vi "Initialize Input DMA Refs.vi"(8 "error in (no error)":errorcluster, 10 "Settings.Compiled":T1 {"IncomingRegisters.Settings"."Register"."Data Type" format="%.0x"; "IncomingRegisters.Refs"."Refs"."Data Reference" format="%.0x"; "OutgoingRegisters.Settings"."Register"."Data Type" format="%.0x"; "OutgoingRegisters.Refs"."Refs"."Data Reference" format="%.0x"; "IncomingDMA.Settings"."DMA.Settings"."DMA Host Buffer" items=["1 Second"=1, "2 Seconds"=2, "5 Seconds"=5, "10 Seconds"=10]; "IncomingDMA.Settings"."DMA.Settings"."dt" format="%#_p"; "IncomingDMA.Settings"."DMA.Settings"."Update Rate" items=["1 Hz"=1, "2 Hz"=2, "5 Hz"=5, "10 Hz"=10]; "OutgoingDMA.Settings"."DMA.Settings"."DMA Host Buffer" items=["1 Second"=1, "2 Seconds"=2, "5 Seconds"=5, "10 Seconds"=10]; "OutgoingDMA.Settings"."DMA.Settings"."dt" format="%#_p"; "OutgoingDMA.Settings"."DMA.Settings"."Update Rate" items=["1 Hz"=1, "2 Hz"=2, "5 Hz"=5, "10 Hz"=10]}, 11 "FPGA Ref":refnum<k20>) -> (0 "error out":errorcluster, 2 "DMA Settings":T15[](array[typedef]) {"DMA Settings"."DMA Host Buffer" items=["1 Second"=1, "2 Seconds"=2, "5 Seconds"=5, "10 Seconds"=10]; "DMA Settings"."dt" format="%#_p"; "DMA Settings"."Update Rate" items=["1 Hz"=1, "2 Hz"=2, "5 Hz"=5, "10 Hz"=10]}, 3 "FPGA Ref":refnum<k20>)   [LabVIEW 2016, in "FPGA Addon Engine.lvlib"]
uses:
  FPGA Addon Engine.lvlib
  Types/DMA Input References.ctl
  <vilib>/NI Veristand/Custom Device Waveform API/Multiple Waveforms Write (DBL)/Multiple Waveforms Write (DBL).lvclass
  Types/DMA Input Ref.ctl
  FPGA-Resource-Manager-APIs/Source/Shared/Types/DMA Settings.ctl
  FPGA-Resource-Manager-APIs/Source/Shared/Types/Delacing Scheme.ctl
  FPGA-Resource-Manager-APIs/Source/Shared/Types/DMA Acquisition Mode.ctl
  FPGA-Resource-Manager-APIs/Source/Shared/Types/Compiled.Settings.ctl
  FPGA-Resource-Manager-APIs/Source/Shared/Types/Compiled.RegisterSettings.ctl
  FPGA-Resource-Manager-APIs/Source/Shared/Types/Scalar Type.ctl
  FPGA-Resource-Manager-APIs/Source/Shared/Types/Register Information.ctl
  FPGA-Resource-Manager-APIs/Source/Shared/Types/Data Type.ctl
  <vilib>/NI Veristand/Custom Device API/Block Data Reference.ctl
  <vilib>/NI Veristand/Custom Device API/Data Reference.ctl
  FPGA-Resource-Manager-APIs/Source/Shared/Types/Compiled.DMASettings.ctl
  <vilib>/NI Veristand/Custom Device API/Waveform Data Reference.ctl
  FPGA-Resource-Manager-APIs/Source/Shared/Types/FPGA Settings.ctl
  <vilib>/NI Veristand/Custom Device API/Custom Device Target Type.ctl
  <vilib>/NI/LVFPGA Adv Session Resources/OpenByNameSubVI.vi
  <vilib>/NI Veristand/Custom Device Waveform API/Multiple Waveforms Write (DBL)/NI VeriStand - Open Multiple Waveforms Write Session (DBL).vi
  <vilib>/Utility/error.llb/Error Cluster From Error Code.vi
  <vilib>/rvi/interface/common/niFpgaWaitOnOcc.vi
  <vilib>/rvi/interface/common/dynamic/niFpgaEscapeDelimiterAndNull.vi
  <vilib>/rvi/interface/nirviMethod/nirviMethod.xnode
  <vilib>/NI/LVFPGA Adv Session Resources/OpenByName.xnode
  <vilib>/NI VeriStand/Custom Device Waveform API/NI_VS Custom Device Waveform API.lvlib
  <vilib>/rvi/errors/niLvFpgaMergeErrorWithErrorCode.vi
  FPGA-Resource-Manager-APIs/Source/Shared/FPGA RM Shared API.lvlib
  <vilib>/FPGAPlugInAG/Dynamic/niLvFpga_ConfigureFifo_Dynamic.vi
  <vilib>/FPGAPlugInAG/Dynamic/niLvFpga_StartFifo_Dynamic.vi
  <vilib>/NI/LVFPGA Adv Session Resources/LVFPGAAdvSessionResources.lvlib
  <vilib>/NI VeriStand/Custom Device API/Custom Device API.lvlib
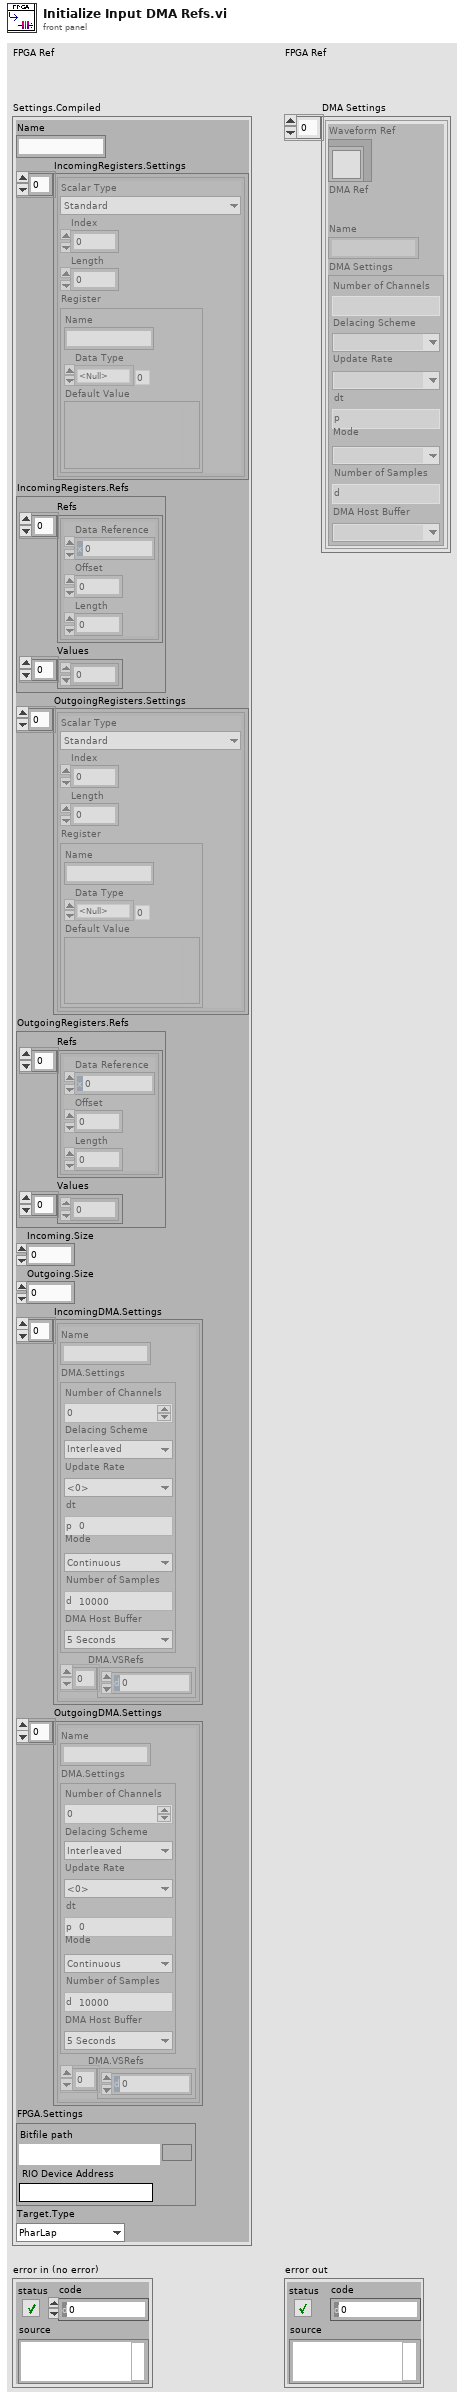
[diagram p1: front panel]
types:
  T1 = typedef "FPGA RM Shared API.lvlib/Compiled.Settings.ctl" = cluster{"Name":string, "IncomingRegisters.Settings":T2[], "IncomingRegisters.Refs":cluster{"Refs":T6[], "Values":dbl[]}, "OutgoingRegisters.Settings":T2[], "OutgoingRegisters.Refs":cluster{"Refs":T6[], "Values":dbl[]}, "Incoming.Size":i32, "Outgoing.Size":i32, "IncomingDMA.Settings":T8[], "OutgoingDMA.Settings":T8[], "FPGA.Settings":T13, "Target.Type":T14}
  T2 = typedef "FPGA RM Shared API.lvlib/Compiled.RegisterSettings.ctl" = cluster{"Scalar Type":T3, "Index":i32, "Length":i32, "Register":T4}
  T3 = typedef "FPGA RM Shared API.lvlib/Scalar Type.ctl" = enum16{"Standard", "Bitpacked"}
  T4 = typedef "FPGA RM Shared API.lvlib/Register Information.ctl" = cluster{"Name":string, "Data Type":T5, "Default Value":variant}
  T5 = typedef "FPGA RM Shared API.lvlib/Data Type.ctl" = enum8{"<Null>", "I8", "I16", "I32", "I64", "U8", "U16", "U32", "U64", "SGL", "Boolean", "Analog PWM In Settings", "Analog PWM In", "Digital PWM In Settings", "Digital PWM In", "Digital PWM Out", "Sine Out", "FXP+/-24.5", "FXP+/-16.5", "FXP+/-32.8", "FXP+/-64.32", "FXP+/-16.7", "FXP+/-20.5"}
  T6 = typedef "Custom Device API.lvlib/Block Data Reference.ctl" = cluster{"Data Reference":T7, "Offset":u64, "Length":u64}
  T7 = typedef "Custom Device API.lvlib/Data Reference.ctl" = i32
  T8 = typedef "FPGA RM Shared API.lvlib/Compiled.DMASettings.ctl" = cluster{"Name":string, "DMA.Settings":T9, "DMA.VSRefs":T12[]}
  T9 = typedef "FPGA RM Shared API.lvlib/DMA Settings.ctl" = cluster{"Number of Channels":u8, "Delacing Scheme":T10, "Update Rate":u32, "dt":dbl, "Mode":T11, "Number of Samples":u32, "DMA Host Buffer":u32}
  T10 = typedef "FPGA RM Shared API.lvlib/Delacing Scheme.ctl" = enum8{"Interleaved"}
  T11 = typedef "FPGA RM Shared API.lvlib/DMA Acquisition Mode.ctl" = enum8{"Continuous", "Triggered Finite"}
  T12 = typedef "Custom Device API.lvlib/Waveform Data Reference.ctl" = i32
  T13 = typedef "FPGA RM Shared API.lvlib/FPGA Settings.ctl" = cluster{"Bitfile path":path, "RIO Device Address":string}
  T14 = typedef "Custom Device API.lvlib/Custom Device Target Type.ctl" = enum16{"PharLap", "VxWorks", "Windows", "Linux_32_ARM", "Linux_x64"}
  T15 = typedef "FPGA Addon Engine.lvlib/DMA Input References.ctl" = cluster{"Waveform Ref":refnum<class "Multiple Waveforms Write (DBL).lvclass">, "DMA Ref":T16, "Name":string, "DMA Settings":T9}
  T16 = typedef "FPGA Addon Engine.lvlib/DMA Input Ref.ctl" = refnum<k20>
  T17 = cluster{"Name":string, "Depth":u32, "Write? (Deprecated:Use Implementation)":bool, "Physical Channel":u32, "Base Address":u32, "Data Width":u32, "Data Type":enum32{"Boolean", "I8", "I16", "I32", "I64", "U8", "U16", "U32", "U64", "FXP", "CustomControl", "SGL"}, "FXP Properties":variant, "Write Window Address":u32, "Implementation":enum16{"niFpgaTargetToHost", "niFpgaHostToTarget", "niFpgaPeerToPeerWriter", "niFpgaPeerToPeerReader", "niCoreTargetToHost", "niCoreHostToTarget"}, "Control Set":u32}[]
  T18 = cluster{"Name":string, "type":variant, "indicator?":bool}[]
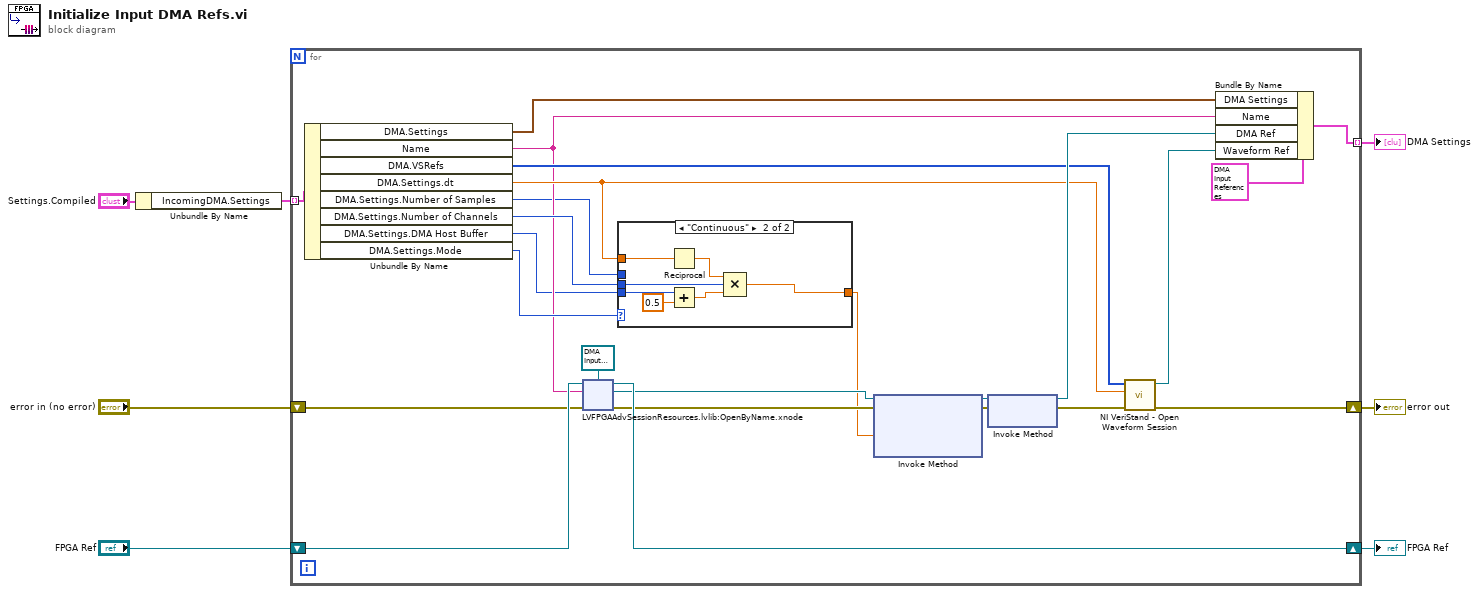
[diagram p0: block diagram]
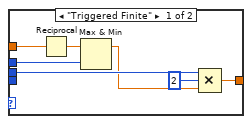
[diagram p2: hidden frame]
diagram:
  n1 = Unbundle By Name("Settings.Compiled") -> ("IncomingDMA.Settings"=w3:T8[])
  n2 = for {
    shift-right: [w29] -> w6
    shift-left: "FPGA Ref" -> [w30]
    tunnel: [w28] -> w5 mode=indexing
    tunnel: w3 -> [w20] mode=indexing
    shift-right: [w9] -> w2
    shift-left: "error in (no error)" -> [w18]
    n3 = Unbundle By Name(w20) -> ("DMA.Settings"=w13:T9, "Name"=w11:string, "DMA.VSRefs"=w17:T12[], "DMA.Settings.dt"=w21:dbl, "DMA.Settings.Number of Samples"=w10:u32, "DMA.Settings.Number of Channels"=w15:u8, "DMA.Settings.DMA Host Buffer"=w8:u32, "DMA.Settings.Mode"=w12:T11)
    n4 = xnode "LVFPGAAdvSessionResources.lvlib:OpenByName.xnode"("FPGA VI Reference in"=w30, "Resource name in"=w11, "Single resource reference type in"=T16 refnum, "Error in"=w18) -> ("Single resource reference out"=w24:T16, "Error out"=w25:errorcluster, "FPGA VI Reference out"=w29:refnum<k20>)
    n5 = case shown="\"Continuous\"" w12 {
      tunnel: [w36 w45] -> w22
      tunnel: w21 -> [w35 w44]
      tunnel: w15 -> [w37 w43]
      tunnel: w10 -> [w33 _]
      tunnel: w8 -> [_ w42]
      frame "Triggered Finite" {
        n6 = Reciprocal(x=w35) -> (1/x=w34:dbl)
        n7 = Max & Min(x=w34, y=w33) -> (max(x,y)=w32:dbl)  [unwired: 1 out]
        n8 = Compound Arithmetic op=MULTIPLY(w37, u8 2 ("value"), w32) -> (w36:dbl)
      }
      frame "Continuous" {
        n9 = Reciprocal(x=w44) -> (1/x=w39:dbl)
        n10 = Add(x=w42, y=0.5 ("x")) -> (x+y=w41:dbl)
        n11 = Compound Arithmetic op=MULTIPLY(w39, w43, w41) -> (w45:dbl)
      }
    }
    n12 = xnode "Invoke Method"("FPGA VI Reference In"=w24, "error in"=w25, "Requested Depth"=w22) -> ("FPGA VI Reference Out"=w27:T16, "error out"=w26:errorcluster)  [unwired: 1 out]
    n13 = xnode "Invoke Method"("FPGA VI Reference In"=w27, "error in"=w26) -> ("FPGA VI Reference Out"=w23:T16, "error out"=w19:errorcluster)
    n14 = call-poly <vilib>:"NI VeriStand - Open Waveform Session.vi"("error in (no error)"=w19, "dt"=w21, "DBL Waveform Data References"=w17) -> ("error out"=w9:errorcluster, "Multiple Waveforms Write Session (DBL)"=w16:refnum<class "Multiple Waveforms Write (DBL).lvclass">)  [unwired: 7 in]
    n15 = Bundle By Name(cluster=T15 {"Waveform Ref"=refnum, "DMA Ref"=refnum, "Name"="", "DMA Settings"={"Number of Channels"=0, "Delacing Scheme"=enum."Interleaved", "Update Rate"=0, "dt"=0.0, "Mode"=enum."Continuous", "Number of Samples"=10000, "DMA Host Buffer"=5}}, "DMA Settings"=w13, "Name"=w11, "DMA Ref"=w23, "Waveform Ref"=w16) -> (w28:T15)
  }
  "error out" <- w2
  "FPGA Ref" <- w6
  "DMA Settings" <- w5
